vi "Read Output.vi"(8 "error in (no error)":errorcluster, 11 "Power Supply in":refnum<class "Power Supply.lvclass">) -> (0 "error out":errorcluster, 1 "persistent?":bool, 2 "Field":dbl[unit], 3 "Power Supply out":refnum<class "Power Supply.lvclass">)   [LabVIEW 2009, in "Power Supply.lvclass"]
uses:
  Power Supply.lvclass
  Power Supply.lvclass/Power Supply.ctl
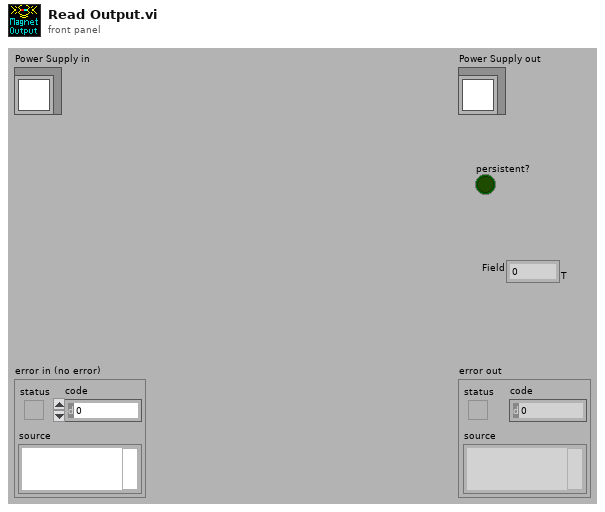
[diagram p1: front panel]
types:
  T1 = typedef "PSIO.ctl" = cluster{"Address":T2, "Version":enum16{"PS", "IPS"}}
  T2 = typedef "OxfordAddress.ctl" = cluster{"Com Port":i32, "ISOBUS Address":i32, "GPIB Address":i16, "Communication":enum16{"RS232", "ISOBUS", "GPIB", "Gateway"}}
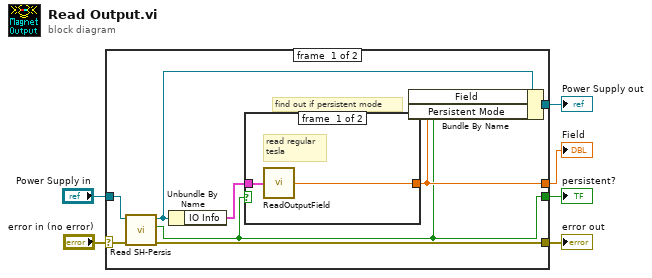
[diagram p0: block diagram]
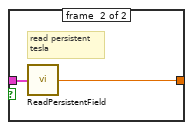
[diagram p2: hidden frame]
diagram:
  n1 = case shown="No Error" "error in (no error)" {
    selector: "error in (no error)" -> [w10 w19]
    tunnel: [w7 _] -> w6
    tunnel: [w8 _] -> w5
    tunnel: "Power Supply in" -> [w14 w20]
    tunnel: [w13 w19] -> w3
    tunnel: [w9 w20] -> w2
    frame #0 {
      # "find out if persistent mode"
      n2 = call-dynamic "Read SH-Persis.vi"("error in (no error)"=w10, "Power Supply in"=w14) -> ("error out"=w13:errorcluster, "pers?"=w7:bool, "Power Supply out"=w12:refnum<class "Power Supply.lvclass">)  [unwired: 4 in, 3 out]
      n3 = Unbundle By Name(w12) -> ("IO Info"=w11:T1)
      n4 = case shown="False" w7 {
        tunnel: w11 -> [w16 w18]
        tunnel: [w15 w17] -> w8
        frame #0 {
          # "read regular\ntesla"
          n5 = call "ReadOutputField.vi"("IO Info"=w16) -> ("Field"=w15:dbl[unit])  [unwired: 2 out]
        }
        frame #1 {
          # "read persistent\ntesla"
          n6 = call "ReadPersistentField.vi"("IO Info"=w18) -> ("Persistent Field"=w17:dbl[unit])  [unwired: 2 out]
        }
      }
      n7 = Bundle By Name(cluster=w12, "Field"=w8, "Persistent Mode"=w7) -> (w9:refnum<class "Power Supply.lvclass">)
    }
    frame #1 {
    }
  }
  "persistent?" <- w6
  "Field" <- w5
  "Power Supply out" <- w2
  "error out" <- w3
